vi "SinAtan2.vi"(10 "X":dbl, 11 "Y":dbl) -> (0 "sec(atan2(x,y))":dbl, 1 "csc(atan2(x,y))":dbl, 2 "cos(atan2(x,y))":dbl, 3 "sin(atan2(x,y))":dbl)   [LabVIEW 2012]
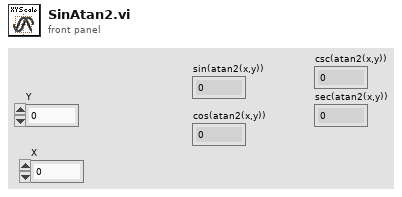
[diagram p1: front panel]
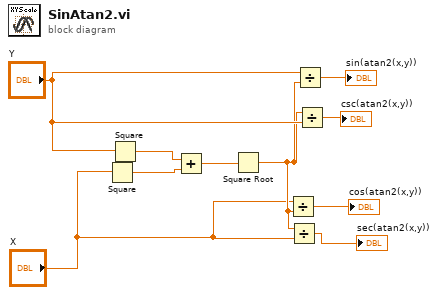
[diagram p0: block diagram]
diagram:
  n1 = Square(x="X") -> (x^2=w7:dbl)
  n2 = Square(x="Y") -> (x^2=w10:dbl)
  n3 = Add(x=w10, y=w7) -> (x+y=w9:dbl)
  n4 = Square Root(x=w9) -> (sqrt(x)=w3:dbl)
  n5 = Divide(x="X", y=w3) -> (x/y=→"cos(atan2(x,y))":dbl)
  n6 = Divide(x=w3, y="X") -> (x/y=→"sec(atan2(x,y))":dbl)
  n7 = Divide(x="Y", y=w3) -> (x/y=→"sin(atan2(x,y))":dbl)
  n8 = Divide(x=w3, y="Y") -> (x/y=→"csc(atan2(x,y))":dbl)
